vi "lab7-adc.vi"() -> ()   [LabVIEW 2018]
uses:
  <vilib>/DAQmx/read.llb/DAQmx Read (Analog 1D DBL 1Chan NSamp).vi
  <vilib>/DAQmx/create/channels.llb/DAQmx Create Channel (AI-Voltage-Basic).vi
  <vilib>/DAQmx/configure/timing.llb/DAQmx Timing (Sample Clock).vi
  <vilib>/DAQmx/miscellaneous.llb/DAQmx Fill In Error Info.vi
  <vilib>/Analysis/NI_AALPro.lvlib
panel:
  out "error out":errorcluster
  out "Fourier spectrum":dbl[](graph)
  in  "source":tag
  out "Waveform Graph":dbl[](graph)
  in  "rate":dbl=1000.0 format="%0.2f"
  in  "samples per channel":i32=1000
  in  "physical channels":tag
  in  "error in":errorcluster
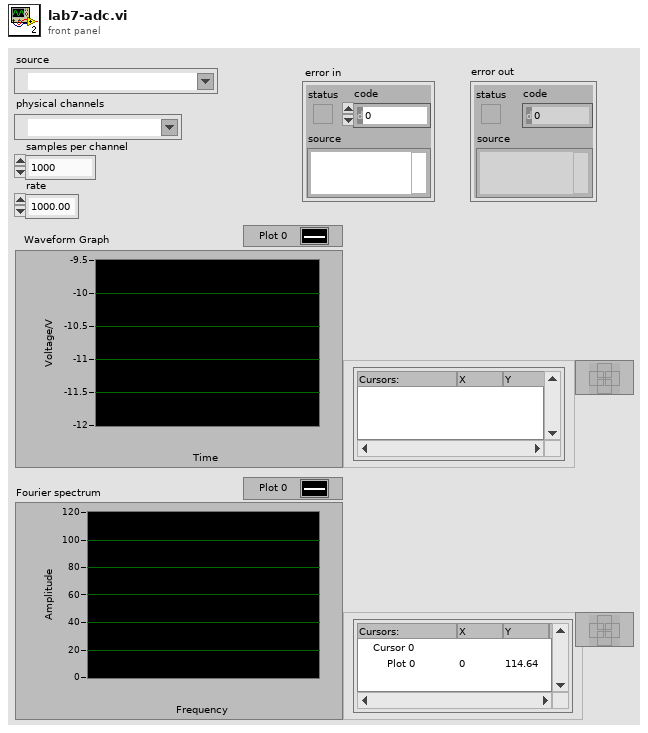
[diagram p1: front panel]
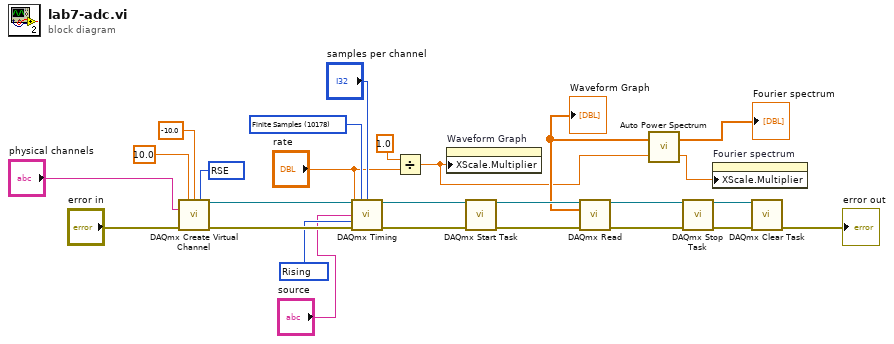
[diagram p0: block diagram]
diagram:
  w12 = 10083 items=["Default"=-1, "RSE"=10083, "NRSE"=10078, "Differential"=10106, "Pseudodifferential"=12529] ("input terminal configuration")
  w11 = 10280 items=["Rising"=10280, "Falling"=10171] ("active edge")
  w23 = 10178 items=["Finite Samples"=10178, "Continuous Samples"=10123, "Hardware Timed Single Point"=12522] ("sample mode")
  n1 = call-poly <vilib>:"DAQmx Create Virtual Channel.vi"("maximum value"=10.0, "minimum value"=-10.0, "input terminal configuration"=w12, "physical channels"="physical channels", "error in"="error in") -> ("task out"=w25:refnum<k21>, "error out"=w24:errorcluster)  [unwired: 9 in]
  n2 = call-poly <vilib>:"DAQmx Timing.vi"("task/channels in"=w25, "sample mode"=w23, "samples per channel"="samples per channel", "rate"="rate", "source"="source", "active edge"=w11, "error in"=w24) -> ("task out"=w22:refnum<k21>, "error out"=w21:errorcluster)  [unwired: 7 in]
  n3 = Divide(x=1.0, y="rate") -> (x/y=w6:dbl)
  n4 = property on="Waveform Graph" class="WFGraph (strict)"("XScale.Multiplier"=w6) -> ()  [unwired: 2 in, 2 out]
  n5 = call <vilib>:"DAQmx Start Task.vi"("task/channels in"=w22, "error in"=w21) -> ("task out"=w16:refnum<k21>, "error out"=w2:errorcluster)  [unwired: 12 in]
  n6 = call-poly <vilib>:"DAQmx Read.vi"("task/channels in"=w16, "error in"=w2) -> ("task out"=w15:refnum<k21>, "data"=w7:dbl[], "error out"=w3:errorcluster)  [unwired: 11 in]
  "Waveform Graph" <- w7
  n7 = call <vilib>:"Auto Power Spectrum.vi"("dt"=w6, "Signal (V)"=w7) -> ("df"=w4:dbl, "Power Spectrum (V^2 rms)"=→"Fourier spectrum":dbl[])
  n8 = call <vilib>:"DAQmx Stop Task.vi"("task/channels in"=w15, "error in"=w3) -> ("task out"=w20:refnum<k21>, "error out"=w19:errorcluster)  [unwired: 12 in]
  n9 = property on="Fourier spectrum" class="WFGraph (strict)"("XScale.Multiplier"=w4) -> ()  [unwired: 2 in, 2 out]
  n10 = call <vilib>:"DAQmx Clear Task.vi"("task in"=w20, "error in"=w19) -> ("error out"=→"error out":errorcluster)  [unwired: 13 in]
